vi "Unflatten (offset).vi"(8 "error in (no error)":errorcluster, 9 "offset (0)":i32, 10 "JSON stream":string, 11 "JSON Value in":refnum<class "JSON Value.lvclass">) -> (0 "error out":errorcluster, 1 "offset":i32, 3 "JSON Value out":refnum<class "JSON Value.lvclass">, 4 "Empty?":bool)   [LabVIEW 2011, in "JSON Value.lvclass"]
doc: "Converts a <b>JSON stream</b> into a <b>JSON Value</b>.\n\nCopyright 2012 James David Powell, Shaun Rumbell and Ton Plomp\nMore information on http://lavag.org/topic/16217-cr-json-labview"
uses:
  JSON Value.lvclass
  JSON Array/JSON Array.lvclass
  JSON Object/JSON Object.lvclass
  JSON Scalar/JSON Scalar.lvclass
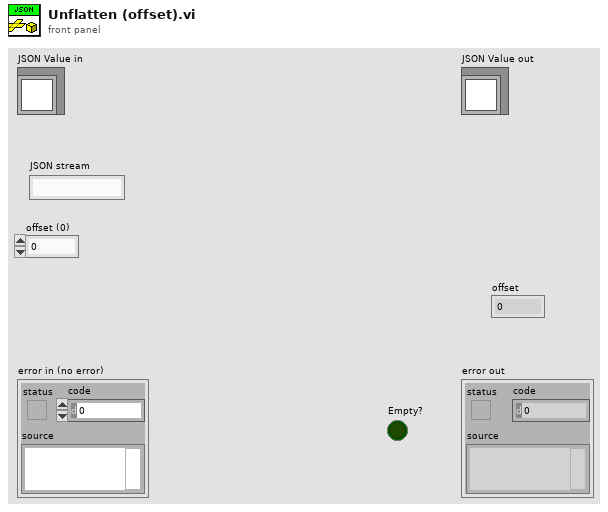
[diagram p1: front panel]
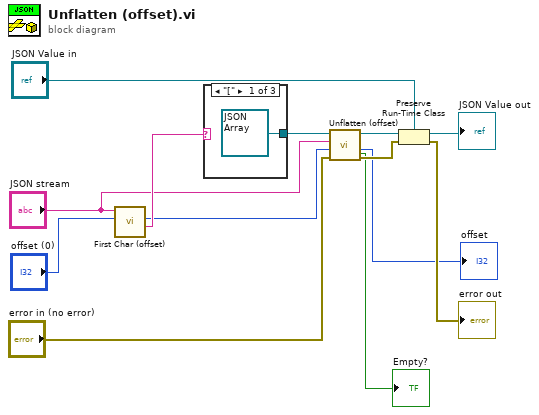
[diagram p0: block diagram]
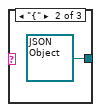
[diagram p2: hidden frame]
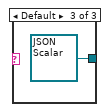
[diagram p3: hidden frame]
diagram:
  n1 = call "First Char (offset).vi"("offset (0)"="offset (0)", "String in"="JSON stream") -> ("First Char"=w4:string, "Offset"=w3:i32)  [unwired: 8 in]
  n2 = case shown="\"[\"" w4 {
    tunnel: [refnum<class "JSON Array.lvclass"> refnum ("JSON Array.lvclass") refnum<class "JSON Object.lvclass"> refnum ("JSON Object.lvclass") refnum<class "JSON Scalar.lvclass"> refnum ("JSON Scalar.lvclass")] -> w10
    frame "[" {
    }
    frame "{" {
    }
    frame Default {
    }
  }
  n3 = call-dynamic "Unflatten (offset).vi"("error in (no error)"="error in (no error)", "offset (0)"=w3, "JSON stream"="JSON stream", "JSON Value in"=w10) -> ("error out"=w9:errorcluster, "offset"=→"offset":i32, "JSON Value out"=w8:refnum<class "JSON Value.lvclass">, "Empty?"=→"Empty?":bool)  [unwired: 4 in]
  n4 = Preserve Run-Time Class(object in=w8, error in=w9, 2:"JSON Value in") -> (object out=→"JSON Value out":refnum<class "JSON Value.lvclass">, error out=→"error out":errorcluster)
